vi "Transmit.vi"(8 "Error In(No Error)":errorcluster, 10 "pSend In":T2[](array[typedef]), 11 "CAN Device In":T1={"Device Type"=20, "Device Index"=0, "CANInd"=0, "Baud(E_U)"=1835016} {"Baud(E_U)" items=["1000Kbps"=393219, "800Kbps"=393220, "500Kbps"=393223, "250Kbps"=1835016, "125Kbps"=1835025, "100Kbps"=1441827, "50Kbps"=1835052, "20Kbps"=1441971, "10Kbps"=1835232, "5Kbps"=1835457]; "Device Type" items=["PCI5121"=1, "PCI9810"=2, "USBCAN1"=3, "USBCAN2"=4, "PCI9820"=5, "PCI5110"=7, "PC104CAN"=11, "CANETUDP"=12, "PCI9840B"=14, "PC104C2"=15, "PCI9820I"=16, "CANETTCP"=17, "PCIE9221"=24, "PCI5010U"=19, "USBCAN_E_U"=20, "USBCAN_2E_U"=21, "PCI5020U"=22, "PCIE9120I"=27, "PCIE9110I"=28, "PCIE9140I"=29, "USBCAN_4E_U"=31, "USBCAN_8E_U"=34]}) -> (0 "Error Out":errorcluster, 1 "Len":u32, 2 "pSend Out":T2[](array[typedef]), 3 "CAN Device Out":T1={"Device Type"=20, "Device Index"=0, "CANInd"=0, "Baud(E_U)"=1835016} {"Baud(E_U)" items=["1000Kbps"=393219, "800Kbps"=393220, "500Kbps"=393223, "250Kbps"=1835016, "125Kbps"=1835025, "100Kbps"=1441827, "50Kbps"=1835052, "20Kbps"=1441971, "10Kbps"=1835232, "5Kbps"=1835457]; "Device Type" items=["PCI5121"=1, "PCI9810"=2, "USBCAN1"=3, "USBCAN2"=4, "PCI9820"=5, "PCI5110"=7, "PC104CAN"=11, "CANETUDP"=12, "PCI9840B"=14, "PC104C2"=15, "PCI9820I"=16, "CANETTCP"=17, "PCIE9221"=24, "PCI5010U"=19, "USBCAN_E_U"=20, "USBCAN_2E_U"=21, "PCI5020U"=22, "PCIE9120I"=27, "PCIE9110I"=28, "PCIE9140I"=29, "USBCAN_4E_U"=31, "USBCAN_8E_U"=34]})   [LabVIEW 2020, in "ZLGCAN.lvclass"]
uses:
  ZLGCAN.lvclass
  VCI_CAN_OBJ.ctl
  Device.ctl
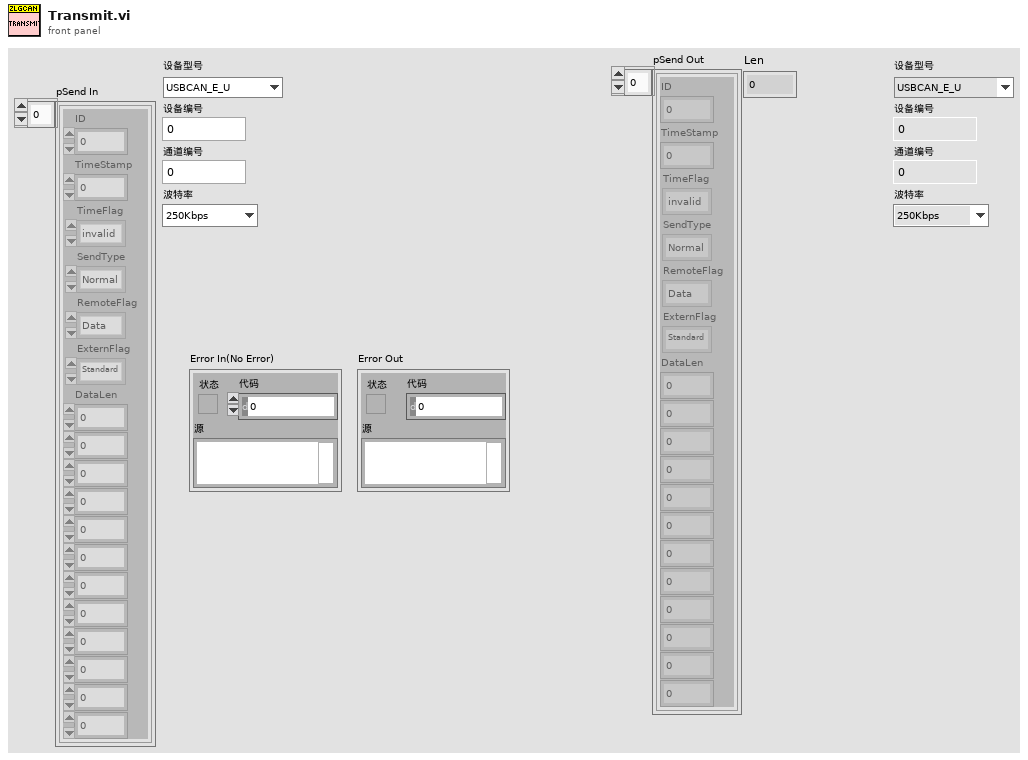
[diagram p1: front panel]
types:
  T1 = typedef "ZLGCAN.lvclass/Device.ctl" = cluster{"Device Type":u32, "Device Index":u32, "CANInd":u32, "Baud(E_U)":u32}
  T2 = typedef "ZLGCAN.lvclass/VCI_CAN_OBJ.ctl" = cluster{"ID":u32, "TimeStamp":u32, "TimeFlag":enum8{"invalid", "valid"}, "SendType":enum8{"Normal", "Once", "Test", "Once Test"}, "RemoteFlag":enum8{"Data", "Remote"}, "ExternFlag":enum8{"Standard", "Extern"}, "DataLen":u8, "Data0":u8, "Data1":u8, "Data2":u8, "Data3":u8, "Data4":u8, "Data5":u8, "Data6":u8, "Data7":u8, "Reserved0":u8, "Reserved1":u8, "Reserved2":u8}
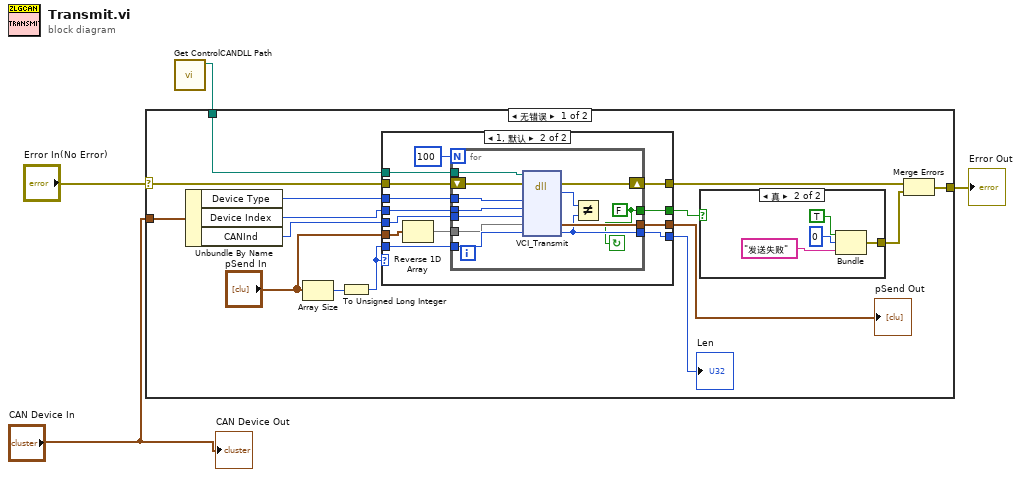
[diagram p0: block diagram]
diagram:
  n1 = call "Get ControlCANDLL Path.vi"() -> ("拆分的路径"=w1:path)  [unwired: 10 in, 1 out]
  n2 = case shown="无错误" "Error In(No Error)" {
    selector: "Error In(No Error)" -> [w19 w50]
    tunnel: [w9 w50] -> w3
    tunnel: "CAN Device In" -> [w17 _]
    tunnel: w1 -> [w6 _]
    frame No Error {
      n3 = Unbundle By Name(w17) -> ("Device Type"=w16:u32, "Device Index"=w15:u32, "CANInd"=w14:u32)
      n4 = Array Size(array="pSend In") -> (size(s)=w13:i32)
      n5 = To Unsigned Long Integer(number=w13) -> (unsigned 32bit integer=w12:u32)
      n6 = case shown="1, 默认" w12 {
        tunnel: [w24 w37] -> w10
        tunnel: [_ w36] -> w5
        tunnel: w19 -> [w24 w35]
        tunnel: "pSend In" -> [_ w30]
        tunnel: w16 -> [_ w34]
        tunnel: w15 -> [_ w33]
        tunnel: w14 -> [_ w32]
        tunnel: w12 -> [_ w31]
        tunnel: [_ w28] -> w8
        tunnel: [_ w27] -> w7
        tunnel: w6 -> [_ w25]
        frame 0 {
        }
        frame 1, Default {
          n7 = Reverse 1D Array(array=w30) -> (reversed array=w29:T2[])
          n8 = for {
            N: 100 -> [_]
            tunnel: [w48] -> w36
            tunnel: w34 -> [w46]
            tunnel: w33 -> [w45]
            tunnel: w32 -> [w44]
            tunnel: w31 -> [w43]
            tunnel: w29 -> [w42]
            tunnel: [w40] -> w28
            tunnel: [w39] -> w27
            shift-right: [w49] -> w37
            shift-left: w35 -> [w47]
            tunnel: w25 -> [w38]
            stop <- w39 continue-if-true
            w39 = FALSE
            n9 = dll-call lib="D:/eDMT Monitor/support/ZLG CAN/ControlCAN.dll" fn="VCI_Transmit"(path in=w38, error in=w47, "DeviceType"=w46, "DeviceInd"=w45, "CANInd"=w44, "pSend"=w42, "Len"=w43) -> (error out=w49:errorcluster, "return type"=w41:u32, "pSend"=w48:T2[], "Len"=w40:u32)  [unwired: 4 in, 1 out]
            n10 = Not Equal?(x=w41, y=w40) -> ()  [unwired: 1 out]
          }
        }
      }
      "pSend Out" <- w5
      "Len" <- w8
      n11 = case shown="真" w7 {
        tunnel: [_ w20] -> w11
        frame False {
        }
        frame True {
          n12 = Bundle("status"=TRUE, "code"=0, "消息"="发送失败") -> (w20:cluster{"status":bool, "code":i32, "消息":string})  [unwired: 1 in]
        }
      }
      n13 = Merge Errors(w10, w11) -> (w9:errorcluster)
    }
    frame Error {
    }
  }
  "Error Out" <- w3
  "CAN Device Out" <- "CAN Device In"
